vi "Check Continuity.vi"(8 "error in (no error)":errorcluster, 11 "Banking Statement in":refnum<class "Banking Statement.lvclass">) -> (0 "error out":errorcluster, 3 "Banking Statement out":refnum<class "Banking Statement.lvclass">)   [LabVIEW 2018, in "Banking Statement.lvclass"]
uses:
  Banking Statement.lvclass
  C:/Users/Jeff Tipps/Documents/Filthy-Lucre-Budgetizer/source/support/classes/Statement/Statement.lvclass
  Statement/Statement.lvclass/Statement.ctl
  <vilib>/Utility/error.llb/DialogType.ctl
  Transaction/Transaction.lvclass
  Statement/Statement.lvclass
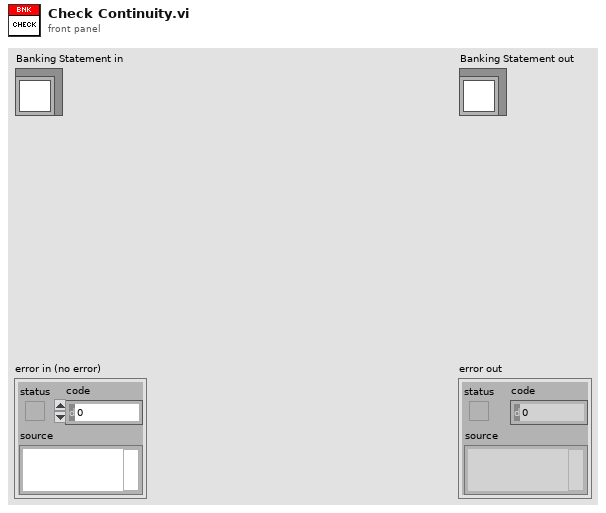
[diagram p1: front panel]
types:
  T1 = typedef "DialogType.ctl" = u16
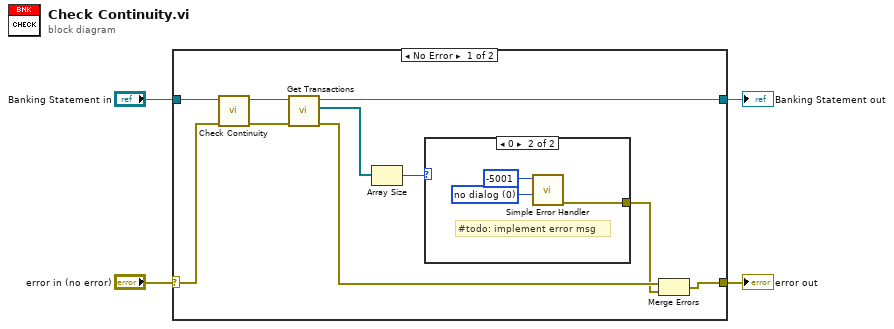
[diagram p0: block diagram]
diagram:
  n1 = case shown="No Error" "error in (no error)" {
    selector: "error in (no error)" -> [w8 w18]
    tunnel: "Banking Statement in" -> [w14 w19]
    tunnel: [w6 w18] -> w3
    tunnel: [w11 w19] -> w2
    frame No Error {
      n2 = call-parent "Check Continuity.vi"("error in (no error)"=w8, "Statement in"=w14) -> ("error out"=w12:errorcluster, "Statement out"=w13:refnum<class "Banking Statement.lvclass">)  [unwired: 8 in]
      n3 = call "Get Transactions.vi"("error in (no error)"=w12, "Statement in"=w13) -> ("error out"=w7:errorcluster, "Transactions"=w10:refnum<class "Transaction.lvclass">[], "Statement out"=w11:refnum<class "Banking Statement.lvclass">)  [unwired: 7 in]
      n4 = Array Size(array=w10) -> (size(s)=w9:i32)
      n5 = case shown="0" w9 {
        tunnel: [_ w15] -> w5
        frame Default {
        }
        frame 0 {
          w16 = T1 0 items=["no dialog", "OK message", "continue or stop message", "OK message + warnings", "continue/stop + warnings"] ("type of dialog (OK msg:1)")
          # "#todo: implement error msg"
          n6 = call <vilib>:"Simple Error Handler.vi"("error code (no error:0)"=-5001, "type of dialog (OK msg:1)"=w16) -> ("error out"=w15:errorcluster)  [unwired: 3 in, 4 out]
        }
      }
      n7 = Merge Errors(w7, w5) -> (w6:errorcluster)
    }
    frame Error {
    }
  }
  "error out" <- w3
  "Banking Statement out" <- w2
